vi "Run Test (Scalar Path).vi"(5 "Test Report":refnum<class "Test Report.lvclass">, 6 "Verbose":bool, 7 "Report Path":path, 8 "error in":errorcluster, 9 "Inspect Recursively (T)":bool=TRUE, 10 "Test Path":path, 11 "Interactive (T)":bool=TRUE) -> (0 "error out":errorcluster)   [LabVIEW 2013, in "Caraya.lvlib"]
uses:
  Caraya.lvlib
  classes/Test Report/Test Report.lvclass
  <userlib>/_OpenG.lib/file/file.llb/Valid Path - Traditional__ogtk.vi
  <userlib>/_OpenG.lib/file/file.llb/File Exists - Scalar__ogtk.vi
  <userlib>/_OpenG.lib/file/file.llb/Strip Path Extension - Path__ogtk.vi
  classes/Test Runner/Test Runner.lvclass
  classes/Test Runner.Folder/Test Runner.Folder.lvclass
  classes/Test Runner.Project/Test Runner.Project.lvclass
  classes/Test Runner.Class/Test Runner.Class.lvclass
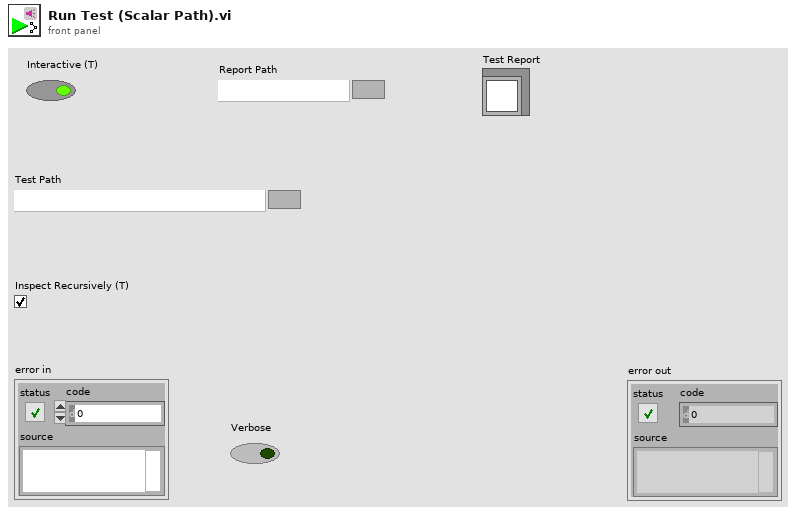
[diagram p1: front panel]
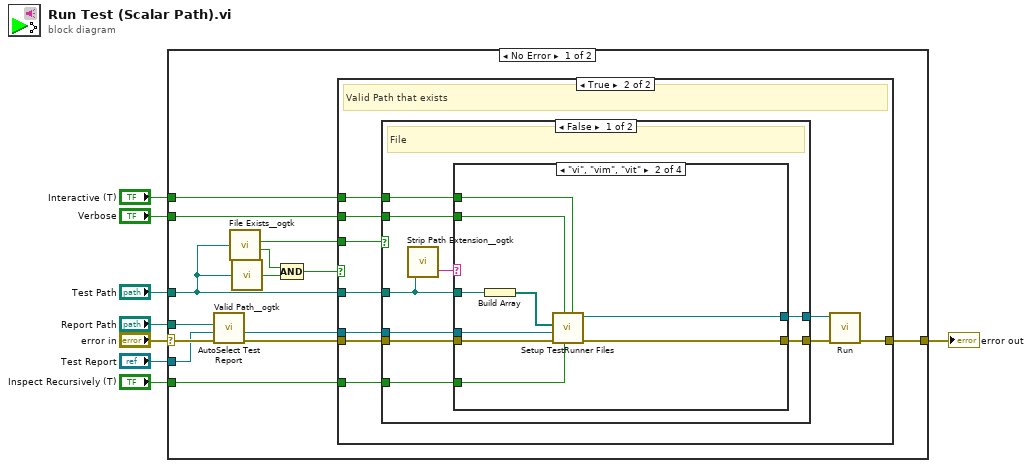
[diagram p0: block diagram]
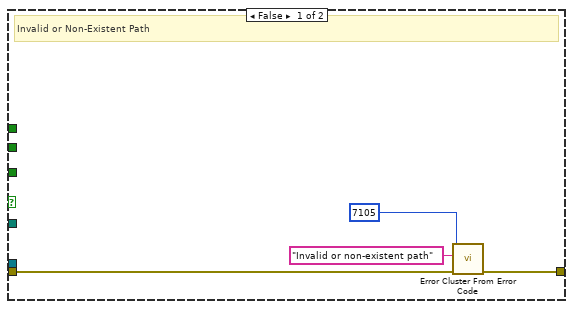
[diagram p2: hidden frame]
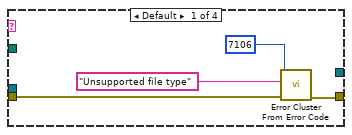
[diagram p3: hidden frame]
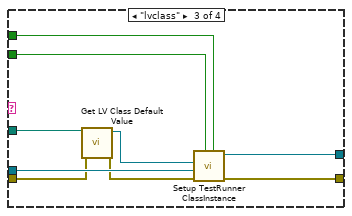
[diagram p4: hidden frame]
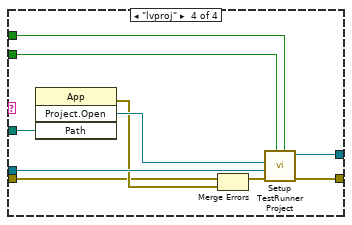
[diagram p5: hidden frame]
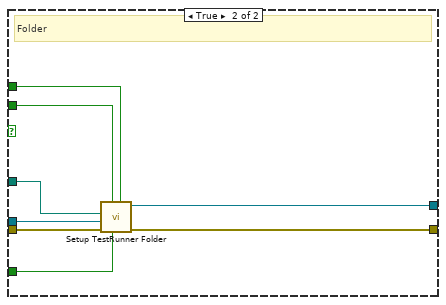
[diagram p6: hidden frame]
diagram:
  n1 = case shown="No Error" "error in" {
    selector: "error in" -> [w19 w86]
    tunnel: [w22 w86] -> w8
    tunnel: "Verbose" -> [w21 _]
    tunnel: "Interactive (T)" -> [w20 _]
    tunnel: "Test Report" -> [w16 _]
    tunnel: "Test Path" -> [w12 _]
    tunnel: "Report Path" -> [w18 _]
    tunnel: "Inspect Recursively (T)" -> [w13 _]
    frame No Error {
      n2 = call "AutoSelect Test Report.vi"("error in (no error)"=w19, "Test Report in"=w16, "Report Path"=w18) -> ("error out"=w17:errorcluster, "Test Report out"=w15:refnum<class "Test Report.lvclass">)  [unwired: 7 in]
      n3 = call-poly <userlib>:"File Exists__ogtk.vi"("file path"=w12) -> ("is directory"=w9:bool, "exists"=w14:bool)  [unwired: 6 in]
      n4 = call-poly <userlib>:"Valid Path__ogtk.vi"("path"=w12) -> ("valid"=w11:bool)
      n5 = Compound Arithmetic op=AND(w14, w11) -> (w10:bool)
      n6 = case shown="True" w10 {
        tunnel: [w25 w36] -> w22
        tunnel: w21 -> [_ w34]
        tunnel: w20 -> [_ w33]
        tunnel: w17 -> [w26 w31]
        tunnel: w15 -> [_ w30]
        tunnel: w13 -> [_ w29]
        tunnel: w12 -> [_ w28]
        tunnel: w9 -> [_ w27]
        frame False {
          # "Invalid or Non-Existent Path"
          n7 = call <vilib>:"Error Cluster From Error Code.vi"("error in (no error)"=w26, "error message (\"\")"="Invalid or non-existent path" ("error message (\"\")"), "error code (0)"=7105 ("code")) -> ("error out"=w25:errorcluster)  [unwired: 6 in]
        }
        frame True {
          # "Valid Path that exists"
          n8 = case shown="False" w27 {
            tunnel: [w44 w85] -> w35
            tunnel: w34 -> [w41 w84]
            tunnel: w33 -> [w42 w83]
            tunnel: [w43 w82] -> w32
            tunnel: w31 -> [w45 w81]
            tunnel: w30 -> [w40 w80]
            tunnel: w28 -> [w38 w79]
            tunnel: w29 -> [w39 w78]
            frame False {
              # "File"
              n9 = call-poly <userlib>:"Strip Path Extension__ogtk.vi"("path"=w38) -> ("extension"=w37:string)  [unwired: 1 out]
              n10 = case shown="\"vi\", \"vim\", \"vit\"" w37 {
                tunnel: w45 -> [w47 w58 w61 w69]
                tunnel: [w46 w57 w67 w76] -> w44
                tunnel: [_ w56 w66 w77] -> w43
                tunnel: w42 -> [_ w55 w65 w73]
                tunnel: w41 -> [_ w54 w64 w74]
                tunnel: w40 -> [_ w53 w63 w75]
                tunnel: w39 -> [_ w52 _ _]
                tunnel: w38 -> [_ w50 w62 w72]
                frame Default {
                  n11 = call <vilib>:"Error Cluster From Error Code.vi"("error in (no error)"=w47, "error message (\"\")"="Unsupported file type" ("error message (\"\")"), "error code (0)"=7106 ("code")) -> ("error out"=w46:errorcluster)  [unwired: 6 in]
                }
                frame "vi", "vim", "vit" {
                  n12 = Build Array(w50) -> (w51:path[])
                  n13 = call "Setup TestRunner Files.vi"("Interactive (T)"=w55, "Inspect Recursively (T)"=w52, "Verbose (F)"=w54, "error in (no error)"=w58, "Test Report"=w53, "Paths"=w51) -> ("error out"=w57:errorcluster, "Test Runner.Folder out"=w56:refnum<class "Test Runner.Folder.lvclass">)  [unwired: 4 in]
                }
                frame "lvclass" {
                  n14 = call <vilib>:"Get LV Class Default Value.vi"("error in (no error)"=w61, "class path"=w62) -> ("error out"=w60:errorcluster, "object"=w59:refnum<class>)  [unwired: 8 in]
                  n15 = call "Setup TestRunner ClassInstance.vi"("Interactive (T)"=w65, "Verbose (F)"=w64, "error in (no error)"=w60, "Test Report"=w63, "Instance"=w59) -> ("error out"=w67:errorcluster, "Test Runner.Class out"=w66:refnum<class "Test Runner.Class.lvclass">)  [unwired: 5 in]
                }
                frame "lvproj" {
                  n16 = invoke class="App" method="Project.Open"("Path"=w72) -> (error out=w70:errorcluster, "Project:Open"=w71:refnum<vi>)  [unwired: 3 in, 2 out]
                  n17 = Merge Errors(w69, w70) -> (w68:errorcluster)
                  n18 = call "Setup TestRunner Project.vi"("Interactive (T)"=w73, "Verbose (F)"=w74, "error in (no error)"=w68, "Test Report"=w75, "Project Refnum"=w71) -> ("error out"=w76:errorcluster, "Test Runner.Project out"=w77:refnum<class "Test Runner.Project.lvclass">)  [unwired: 5 in]
                }
              }
            }
            frame True {
              # "Folder"
              n19 = call "Setup TestRunner Folder.vi"("Interactive (T)"=w83, "Inspect Recursively (T)"=w78, "Verbose (F)"=w84, "error in (no error)"=w81, "Test Report"=w80, "Directory to search"=w79) -> ("error out"=w85:errorcluster, "Test Runner.Folder out"=w82:refnum<class "Test Runner.Folder.lvclass">)  [unwired: 4 in]
            }
          }
          n20 = call "Run.vi"("error in (no error)"=w35, "Test Runner in"=w32) -> ("error out"=w36:errorcluster)  [unwired: 8 in, 1 out]
        }
      }
    }
    frame Error {
    }
  }
  "error out" <- w8
